vi "配置文件路径.vi"() -> (3 "appended path":path)   [LabVIEW 2016, in "斯坦道总磷总氮.lvlib"]
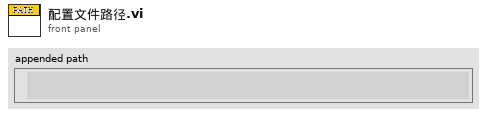
[diagram p1: front panel]
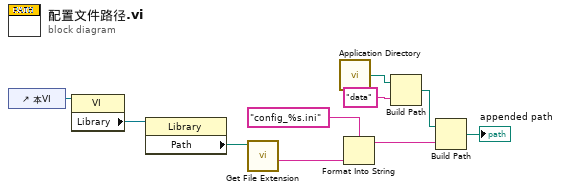
[diagram p0: block diagram]
diagram:
  n1 = control-ref of="本VI"() -> (w7:refnum<vi>)
  n2 = property class="VI"(reference=w7) -> ("Library"=w8:refnum<vi>)  [unwired: 1 in, 2 out]
  n3 = property class="Library"(reference=w8) -> ("Path"=w6:path)  [unwired: 1 in, 2 out]
  n4 = call <vilib>:"Get File Extension.vi"("file"=w6) -> ("filename without extension"=w3:string)  [unwired: 6 in, 4 out]
  n5 = call <vilib>:"Application Directory.vi"() -> ("Application Directory"=w9:path)
  n6 = Format Into String(format string="config_%s.ini" ("格式字符串"), w3) -> (resulting string=w4:string)  [unwired: 2 in, 1 out]
  n7 = Build Path(base path=w9, name or relative path="data" ("名称或相对路径")) -> (appended path=w5:path)
  n8 = Build Path(base path=w5, name or relative path=w4) -> (appended path=→"appended path":path)
